vi "Get UA Numeric Value.vi"(8 "error in (no error)":errorcluster, 10 "Item id in":string, 11 "OPC UA server refnum in":T1) -> (0 "error out":errorcluster, 1 "timestamp out":timestamp, 2 "Item value out":i64, 3 "OPC UA server refnum out":T1)   [LabVIEW 2024, in "OPCUA.lvlib"]
uses:
  <vilib>/OPCUA/controls/OPC UA Server Refnum.ctl
  <vilib>/OPCUA/server/Read Int64.vi
  OPCUA.lvlib
  <vilib>/OPCUA/NI OPC UA Server.lvlib
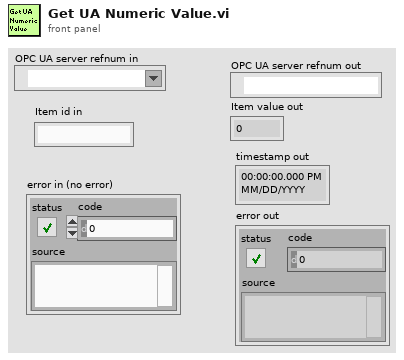
[diagram p1: front panel]
types:
  T1 = typedef "OPC UA Server Refnum.ctl" = refnum<k21>
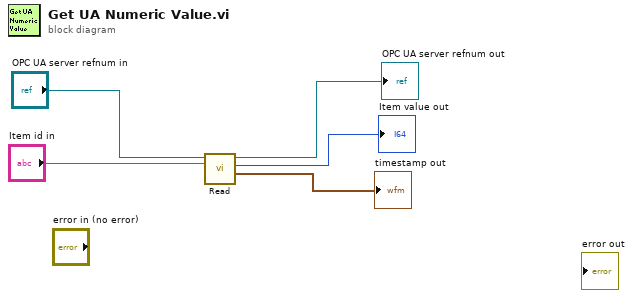
[diagram p0: block diagram]
diagram:
  n1 = call-poly <vilib>:"Read.vi"("node ID"="Item id in", "OPC UA server refnum in"="OPC UA server refnum in") -> ("timestamp"=→"timestamp out":timestamp, "value"=→"Item value out":i64, "OPC UA server refnum out"=→"OPC UA server refnum out":T1)  [unwired: 5 in, 2 out]
